vi "_Current Data Global.vi"(4 "error in (no error)":errorcluster, 5 "AcqMethod":T1[](array[typedef]) {"ScanType" format="%#.6g"; "Mass Range"."Res" items=["High/High", "Medium/Medium", "Low/Low", "High/Medium", "High/Low", "Medium/High", "Medium/Low", "Low/High", "Low/Medium"]}, 6 "Spectrum in":i32[](array[numeric]), 7 "Operation":T7=enum."Get Data") -> (0 "error out":errorcluster, 2 "Latest Raw Data":i32[](array[numeric]), 3 "CurrentData":T6[](array[typedef]) {"Method"."Mass Range"."Res" items=["High/High", "Medium/Medium", "Low/Low", "High/Medium", "High/Low", "Medium/High", "Medium/Low", "Low/High", "Low/Medium"]})   [LabVIEW 2015]
uses:
  Type/_Data Operation.ctl
  Type/_Current Data.ctl
  Type/_XML Expt.ctl
  Type/_XML Lens.ctl
  Type/_Mass Range Property.ctl
  Type/_Mass Range Parameters.ctl
  Type/_RT Res Type.ctl
  Type/_Run Module.ctl
  Type/_File Command.ctl
  Configuration/_Global Configuration.vi
panel:
  # "Raw Data:\nExpt#, Run Time in mS, data array in counts"
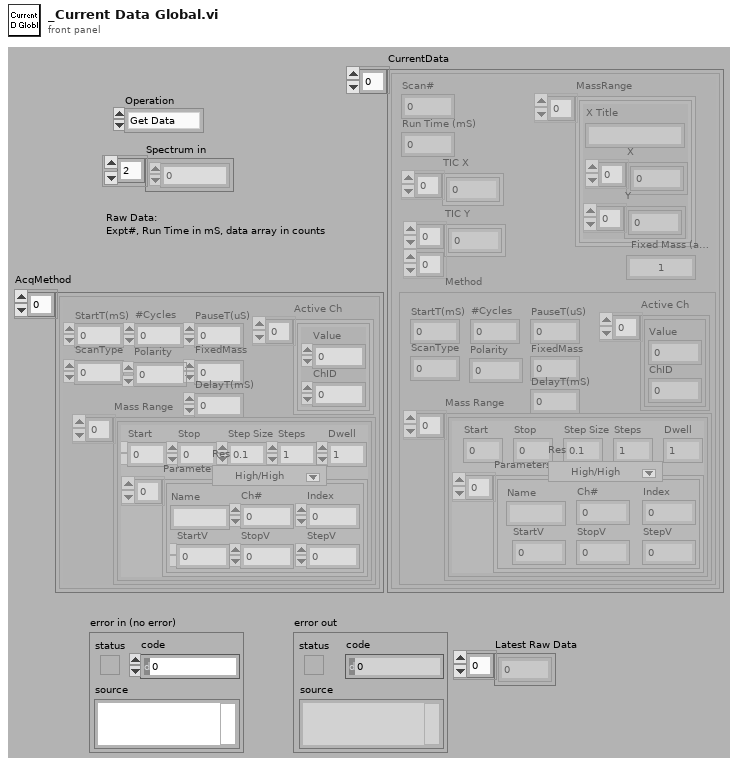
[diagram p1: front panel]
types:
  T1 = typedef "_XML Expt.ctl" = cluster{"StartT(mS)":i32, "#Cycles":i32, "PauseT(uS)":i32, "ScanType":i32, "Polarity":u8, "FixedMass":dbl, "DelayT(mS)":i32, "Active Ch":T2[], "Mass Range":T3[]}
  T2 = typedef "_XML Lens.ctl" = cluster{"Value":dbl, "ChID":u8}
  T3 = typedef "_Mass Range Property.ctl" = cluster{"Start":dbl, "Stop":dbl, "Step Size":dbl, "Steps":i32, "Dwell":dbl, "Parameters":T4[], "Res":T5}
  T4 = typedef "_Mass Range Parameters.ctl" = cluster{"Name":string, "Ch#":u8, "StartV":dbl, "StopV":dbl, "StepV":dbl, "Index":u8}
  T5 = typedef "_RT Res Type.ctl" = u16
  T6 = typedef "_Current Data.ctl" = cluster{"Scan#":i32, "Run Time (mS)":i32, "TIC X":dbl[], "TIC Y":dbl[][], "MassRange":cluster{"X Title":string, "X":dbl[], "Y":i32[]}[], "Fixed Mass (amu)":dbl, "Method":T1}
  T7 = typedef "_Data Operation.ctl" = enum8{"Initialize", "Get Data", "Set Data", "Close"}
  T8 = typedef "_Run Module.ctl" = u16
  T9 = typedef "_File Command.ctl" = enum16{"No Command", "Open", "Open Read", "Write", "Get Spectrum", "Close"}
  T10 = typedef "_Lens Property.ctl" = cluster{"Scan Type":u8, "Scans":i32, "Time 1":dbl, "Time 2":dbl, "Value 1":dbl, "Value 2":dbl, "Step Size":dbl}
  T11 = typedef "_Run Mode.ctl" = enum16{"MRM (Q1/Q2)", "Q1 Scan", "Q1 SRM", "Q2 Scan", "Q2 SRM", "Product Scan", "Precursor Scan", "Neutral Loss", "Neutral Gain"}
  T12 = cluster{"Lenses":T10[], "Mass Ranges":T3[], "Acquire":bool, "MCA":bool, "Q1DC EN":bool, "Q1 POL":bool, "Q3 POL":bool, "Q1 RF  EN":bool, "Averaging":bool, "Log Scale":bool, "CPS":bool, "Unit":bool, "Data Path":path, "Run Mode":T11, "Fixed Mass (amu)":dbl, "Q3DC EN":bool, "Q3 RF  EN":bool, "Negative":bool}
  T13 = cluster{"X Title":string, "X":dbl[], "Y":i32[]}[]
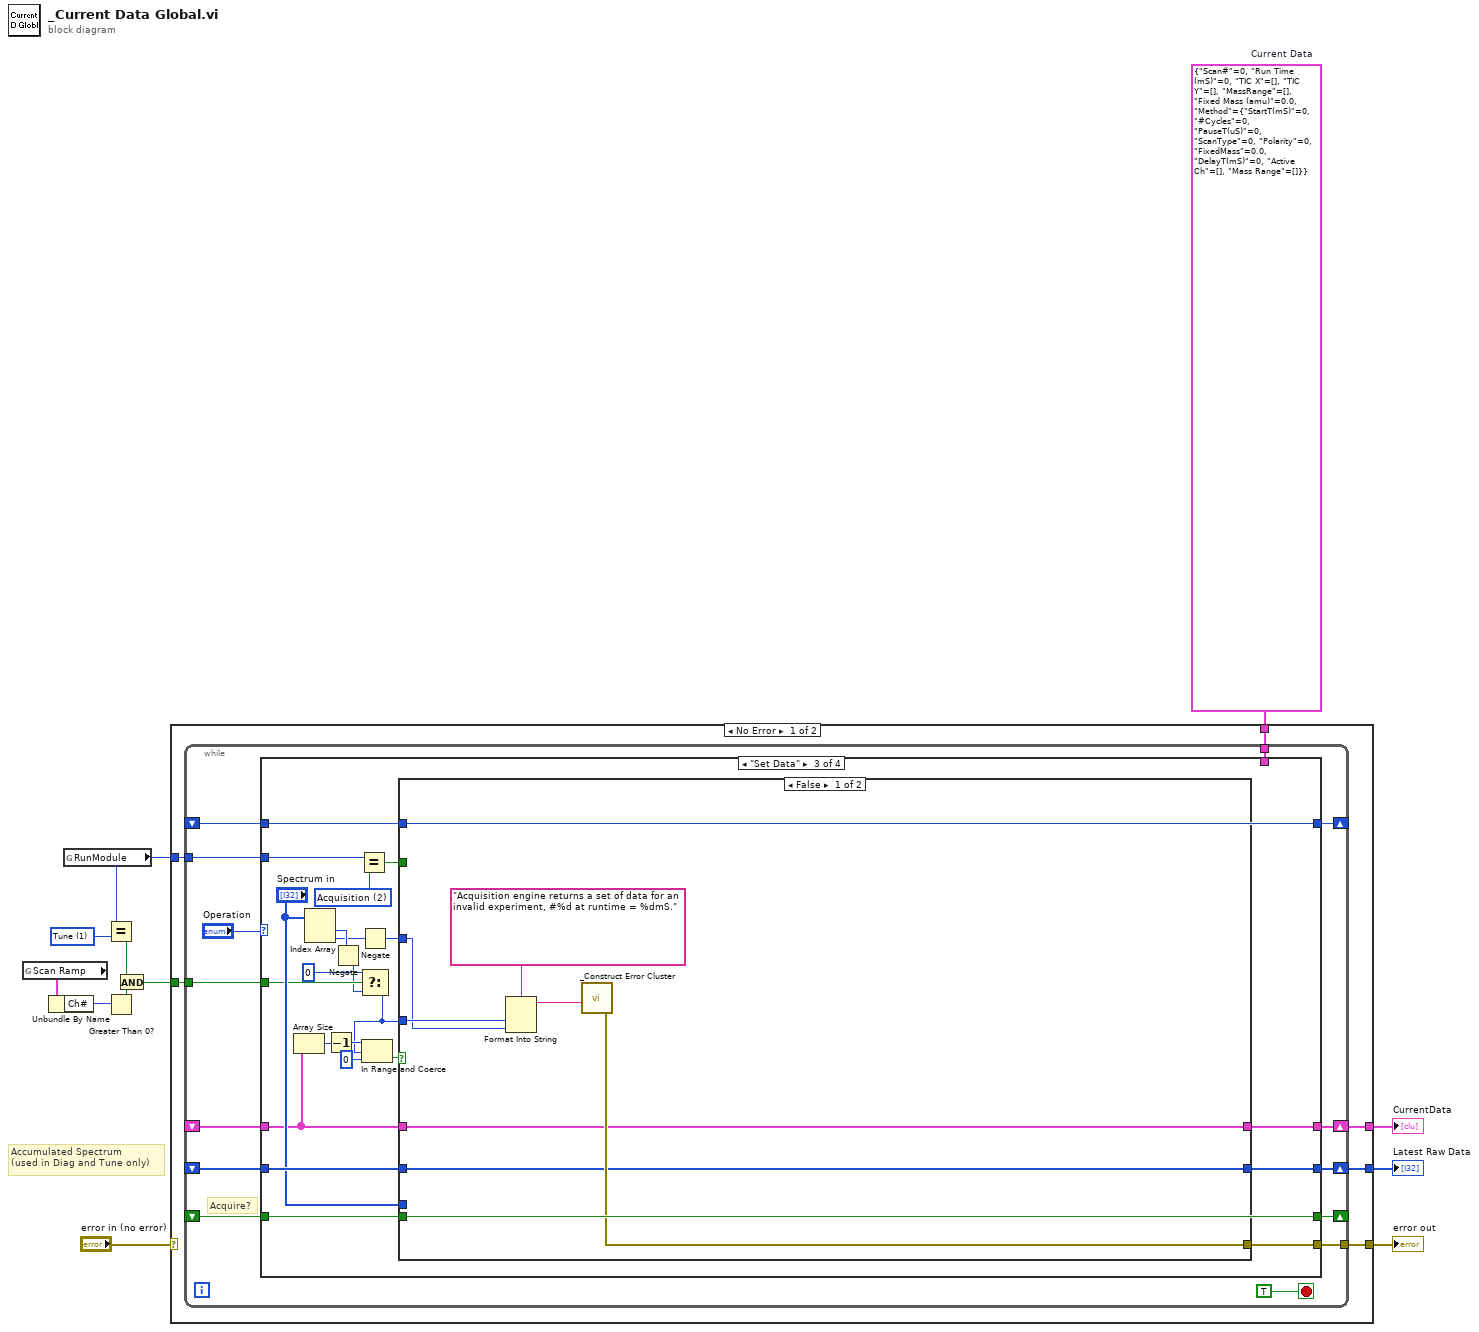
[diagram p0: block diagram]
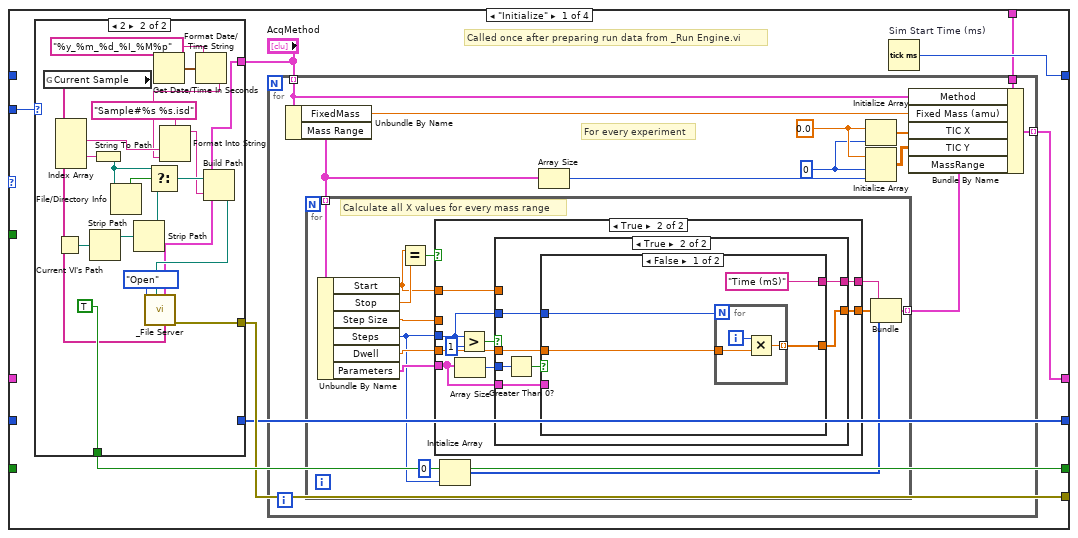
[diagram p2: hidden frame]
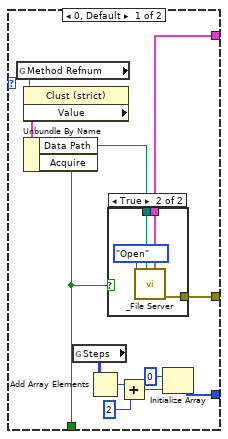
[diagram p3: hidden frame]
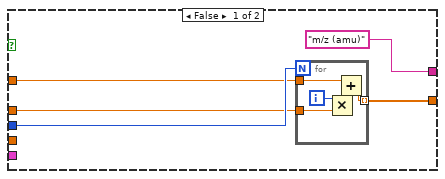
[diagram p5: hidden frame]
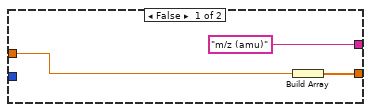
[diagram p6: hidden frame]
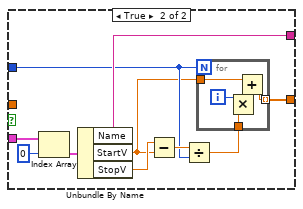
[diagram p7: hidden frame]
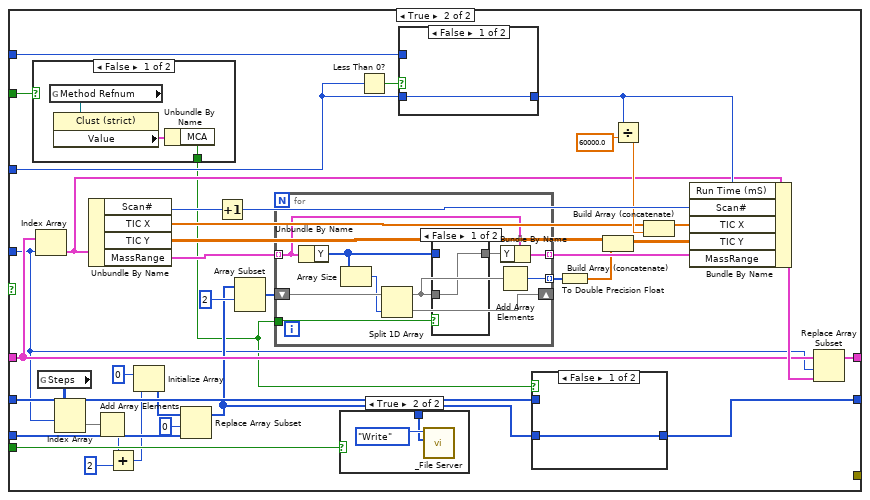
[diagram p9: hidden frame]
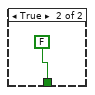
[diagram p10: hidden frame]
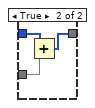
[diagram p11: hidden frame]
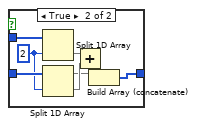
[diagram p12: hidden frame]
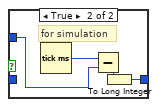
[diagram p14: hidden frame]
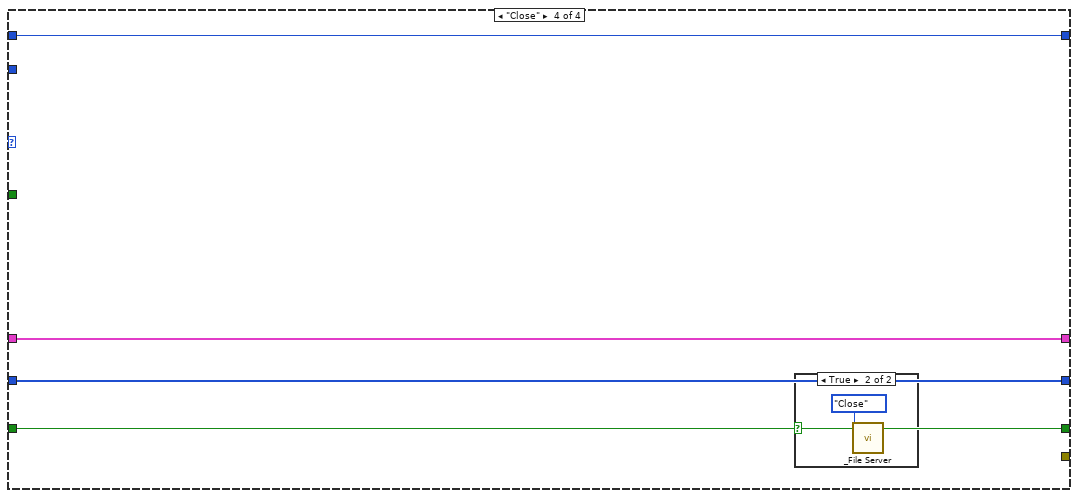
[diagram p15: hidden frame]
diagram:
  w7 = T8 1 items=["Diagnostics", "Tune", "Acquisition"] ("y")
  w9 = T6 {"Scan#"=0, "Run Time (mS)"=0, "TIC X"=[], "TIC Y"=[], "MassRange"=[], "Fixed Mass (amu)"=0.0, "Method"={"StartT(mS)"=0, "#Cycles"=0, "PauseT(uS)"=0, "ScanType"=0, "Polarity"=0, "FixedMass"=0.0, "DelayT(mS)"=0, "Active Ch"=[], "Mass Range"=[]}}  # Current Data
  # "Accumulated Spectrum\n(used in Diag and Tune only)"
  n1 = global read "_Global Configuration.vi" "Scan Ramp"() -> (w6:T4)
  n2 = Unbundle By Name(w6) -> ("Ch#"=w5:u8)
  n3 = global read "_Global Configuration.vi" "RunModule"() -> (w2:T8)
  n4 = Equal?(x=w2, y=w7) -> (x = y?=w4:bool)
  n5 = Greater Than 0?(x=w5) -> (x > 0?=w3:bool)
  n6 = And(x=w4, y=w3) -> (x .and. y?=w1:bool)
  n7 = case shown="No Error" "error in (no error)" {
    selector: "error in (no error)" -> [_ w261]
    tunnel: [w18 _] -> w8
    tunnel: [w17 w261] -> w11
    tunnel: [w16 _] -> w10
    tunnel: w2 -> [w15 _]
    tunnel: w9 -> [w14 _]
    tunnel: w1 -> [w13 _]
    frame No Error {
      n8 = while {
        shift-right: [w30] -> w18
        shift-left: _ -> [w29]
        tunnel: [w28] -> w17
        shift-right: [w27] -> _
        shift-left: _ -> [w26]
        shift-right: [w25] -> w16
        shift-left: _ -> [w24]
        shift-right: [w23] -> _
        shift-left: _ -> [w22]
        tunnel: w15 -> [w21]
        tunnel: w14 -> [w20]
        tunnel: w13 -> [w19]
        stop <- TRUE stop-if-true
        # "Acquire?"
        n9 = case shown="\"Set Data\"" "Operation" {
          tunnel: [w37 w154 w176 w259] -> w30
          tunnel: w29 -> [_ w154 w162 w259]
          tunnel: [w35 _ w165 _] -> w28
          tunnel: [w36 w153 w172 w258] -> w27
          tunnel: w26 -> [_ w153 w172 w258]
          tunnel: [w34 w152 w173 w257] -> w25
          tunnel: w24 -> [_ w152 w174 w257]
          tunnel: [w40 w151 w175 w256] -> w23
          tunnel: w22 -> [_ w151 w175 w256]
          tunnel: w21 -> [w39 _ w161 _]
          tunnel: w20 -> [w38 _ _ _]
          tunnel: w19 -> [_ _ w158 _]
          frame "Initialize" {
            # "Called once after preparing run data from _Run Engine.vi"
            n10 = case shown="2" w39 {
              tunnel: [w49 w72] -> w35
              tunnel: [w48 TRUE] -> w36
              tunnel: [w42 _] -> w34
              tunnel: "AcqMethod" -> [w41 w58]
              frame 0, Default {
                n11 = global read "_Global Configuration.vi" "Method Refnum"() -> (w52:refnum<vi>)
                n12 = property class="Clust (strict)"(reference=w52) -> ("Value"=w51:T12)  [unwired: 1 in, 2 out]
                n13 = Unbundle By Name(w51) -> ("Data Path"=w50:path, "Acquire"=w48:bool)
                n14 = global read "_Global Configuration.vi" "Steps"() -> (w46:i32[][])
                n15 = Add Array Elements(numeric array=w46) -> (sum=w47:i32)
                n16 = case shown="True" w48 {
                  tunnel: [_ w55] -> w49
                  tunnel: w50 -> [_ w54]
                  tunnel: w41 -> [_ w53]
                  frame False {
                  }
                  frame True {
                    n17 = call "_File Server.vi"("AcqMethod"=w53, "file path"=w54, "File Command"=_File_Command."Open") -> ("error out"=w55:errorcluster)  [unwired: 4 in, 4 out]
                  }
                }
                n18 = Add(x=w47, y=2) -> (x+y=w44:i32)
                n19 = Initialize Array(0 ("element"), w44) -> (w42:i32[])
              }
              frame 2 {
                n20 = global read "_Global Configuration.vi" "Current Sample"() -> (w57:string[])
                n21 = Current VI's Path() -> (path=w67:path)
                n22 = Index Array(array=w57) -> (element #1=w71:string, element #3=w75:string)  [unwired: 4 in, 2 out]
                n23 = Strip Path(path=w67) -> (stripped path=w68:path)  [unwired: 1 out]
                n24 = String To Path(string=w75) -> (path=w69:path)
                n25 = File/Directory Info(path=w69) -> (directory=w70:bool)  [unwired: 1 in, 6 out]
                n26 = Strip Path(path=w68) -> (stripped path=w66:path)  [unwired: 1 out]
                n27 = Select(t=w69, s=w70, f=w66) -> (s? t:f=w65:path)
                n28 = Get Date/Time In Seconds() -> (seconds since 1Jan1904=w63:timestamp)
                n29 = Format Date/Time String(time format string (%c)="%y_%m_%d_%I_%M%p", seconds (now)=w63) -> (date/time string=w61:string)  [unwired: 1 out]
                n30 = Format Into String(format string="Sample#%s %s.isd", w71, w61) -> (resulting string=w59:string)  [unwired: 2 in, 1 out]
                n31 = Build Path(base path=w65, name or relative path=w59) -> (appended path=w64:path)
                n32 = call "_File Server.vi"("Sample Info"=w57, "AcqMethod"=w58, "file path"=w64, "File Command"=_File_Command."Open") -> ("error out"=w72:errorcluster)  [unwired: 3 in, 4 out]
              }
            }
            n33 = for {
              tunnel: "AcqMethod" -> [w77] mode=indexing
              tunnel: w38 -> [w86]
              tunnel: [w78] -> w37 mode=indexing
              w81 = 0.0 ("element")
              w76 = 0 ("dimension size")
              # "For every experiment"
              n34 = Unbundle By Name(w77) -> ("FixedMass"=w85:dbl, "Mass Range"=w82:T3[])
              n35 = for {
                tunnel: w82 -> [w99] mode=indexing
                tunnel: [w90] -> w84 mode=indexing
                # "Calculate all X values for every mass range"
                n36 = Unbundle By Name(w99) -> ("Start"=w96:dbl, "Stop"=w97:dbl, "Step Size"=w95:dbl, "Steps"=w87:i32, "Dwell"=w88:dbl, "Parameters"=w89:T4[])
                n37 = Equal?(x=w96, y=w97) -> (x = y?=w98:bool)
                n38 = case shown="True" w98 {
                  tunnel: w87 -> [w104 w111]
                  tunnel: w96 -> [w103 w116]
                  tunnel: w95 -> [w102 _]
                  tunnel: [w101 w114] -> w92
                  tunnel: ["m/z (amu)" ("X Title") w115] -> w93
                  tunnel: w89 -> [_ w110]
                  tunnel: w88 -> [_ w112]
                  frame False {
                    n39 = for {
                      N: w104 -> [_]
                      tunnel: w102 -> [w108]
                      tunnel: w103 -> [w106]
                      tunnel: [w105] -> w101 mode=indexing
                      i -> [w109]
                      n40 = Multiply(x=w109, y=w108) -> (x*y=w107:dbl)
                      n41 = Add(x=w106, y=w107) -> (x+y=w105:dbl)
                    }
                  }
                  frame True {
                    n42 = Array Size(array=w110) -> (size(s)=w113:i32)
                    n43 = Greater?(x=w111, y=1) -> (0:w117:bool)
                    n44 = case shown="True" w117 {
                      tunnel: w116 -> [w119 _]
                      tunnel: ["m/z (amu)" ("X Title") w126] -> w115
                      tunnel: [w120 w123] -> w114
                      tunnel: w113 -> [_ w128]
                      tunnel: w112 -> [_ w125]
                      tunnel: w111 -> [_ w124]
                      tunnel: w110 -> [_ w122]
                      frame False {
                        n45 = Build Array(w119) -> (w120:dbl[])
                      }
                      frame True {
                        n46 = Greater Than 0?(x=w128) -> (x > 0?=w127:bool)
                        n47 = case shown="False" w127 {
                          tunnel: ["Time (mS)" ("X Title") w142] -> w126
                          tunnel: w125 -> [w131 _]
                          tunnel: w124 -> [w130 w139]
                          tunnel: [w129 w136] -> w123
                          tunnel: w122 -> [_ w145]
                          frame False {
                            n48 = for {
                              N: w130 -> [_]
                              tunnel: w131 -> [w134]
                              tunnel: [w133] -> w129 mode=indexing
                              i -> [w135]
                              n49 = Multiply(x=w135, y=w134) -> (x*y=w133:dbl)
                            }
                          }
                          frame True {
                            n50 = Index Array(array=w145, index=0) -> (element=w143:T4)
                            n51 = Unbundle By Name(w143) -> ("Name"=w142:string, "StartV"=w138:dbl, "StopV"=w141:dbl)
                            n52 = Subtract(x=w141, y=w138) -> (x-y=w140:dbl)
                            n53 = Divide(x=w140, y=w139) -> (x/y=w137:dbl)
                            n54 = for {
                              N: w139 -> [_]
                              tunnel: w138 -> [w148]
                              tunnel: [w147] -> w136 mode=indexing
                              tunnel: w137 -> [w146]
                              i -> [w150]
                              n55 = Multiply(x=w150, y=w146) -> (x*y=w149:dbl)
                              n56 = Add(x=w148, y=w149) -> (x+y=w147:dbl)
                            }
                          }
                        }
                      }
                    }
                  }
                }
                n57 = Initialize Array(0 ("element"), w87) -> (w91:i32[])
                n58 = Bundle("Name"=w93, w92, w91) -> (w90:cluster{"Name":string, dbl[], i32[]})  [unwired: 1 out]
              }
              n59 = Array Size(array=w82) -> (size(s)=w83:i32)
              n60 = Initialize Array(w81, w76) -> (w80:dbl[])
              n61 = Initialize Array(w81, w76, w83) -> (w79:dbl[][])
              n62 = Bundle By Name(cluster=w86, "Method"=w77, "Fixed Mass (amu)"=w85, "TIC X"=w80, "TIC Y"=w79, "MassRange"=w84) -> (w78:T6)
            }
            n63 = Tick Count (ms) "Sim Start Time (ms)"() -> (millisecond timer value=w40:u32)
          }
          frame "Get Data", Default {
          }
          frame "Set Data" {
            w160 = T8 2 items=["Diagnostics", "Tune", "Acquisition"] ("y")
            n64 = Array Size(array=w162) -> (size(s)=w169:i32)
            n65 = Index Array(array="Spectrum in") -> (element #1=w170:i32, element #2=w164:i32)  [unwired: 2 in]
            n66 = Decrement(x=w169) -> (x-1=w167:i32)
            n67 = Negate(x=w170) -> (-x=w157:i32)
            n68 = Equal?(x=w161, y=w160) -> (x = y?=w159:bool)
            n69 = Negate(x=w164) -> (-x=w163:i32)
            n70 = Select(t=0, s=w158, f=w157) -> (s? t:f=w155:i32)
            n71 = In Range and Coerce(upper limit=w167, x=w155, lower limit=0) -> (In Range?=w166:bool)  [unwired: 1 out]
            n72 = case shown="False" w166 {
              tunnel: w163 -> [w179 w199]
              tunnel: [w178 w195] -> w176
              tunnel: w175 -> [_ w221]
              tunnel: w174 -> [w177 w220]
              tunnel: [w177 w219] -> w173
              tunnel: w172 -> [_ w218]
              tunnel: "Spectrum in" -> [_ w217]
              tunnel: w155 -> [w183 w192]
              tunnel: [w180 _] -> w165
              tunnel: w162 -> [w178 w196]
              tunnel: w159 -> [_ w185]
              frame False {
                n73 = Format Into String(format string="Acquisition engine returns a set of data for an invalid experiment, #%d at runtime = %dmS.", w183, w179) -> (resulting string=w181:string)  [unwired: 2 in, 1 out]
                n74 = call "_Construct Error Cluster.vi"("reason"=w181) -> ("error out"=w180:errorcluster)  [unwired: 3 in, 3 out]
              }
              frame True {
                n75 = case shown="False" w185 {
                  tunnel: [w222 FALSE] -> w184
                  frame False {
                    n76 = global read "_Global Configuration.vi" "Method Refnum"() -> (w223:refnum<vi>)
                    n77 = property class="Clust (strict)"(reference=w223) -> ("Value"=w224:T12)  [unwired: 1 in, 2 out]
                    n78 = Unbundle By Name(w224) -> ("MCA"=w222:bool)
                  }
                  frame True {
                  }
                }
                n79 = Index Array(array=w196, index=w192) -> (element=w198:T6)
                n80 = global read "_Global Configuration.vi" "Steps"() -> (w193:i32[][])
                n81 = Index Array(array=w193, index (row)=w192) -> (element=w191:i32[])  [unwired: 1 in]
                n82 = Unbundle By Name(w198) -> ("Scan#"=w215:i32, "TIC X"=w209:dbl[], "TIC Y"=w202:dbl[][], "MassRange"=w206:T13)
                n83 = Add Array Elements(numeric array=w191) -> (sum=w190:i32)
                n84 = Add(x=w190, y=2) -> (x+y=w188:i32)
                n85 = Initialize Array(0 ("element"), w188) -> (w186:i32[])
                n86 = Replace Array Subset(array=w186, new element=w217, index=0) -> (w194:i32[])
                n87 = Increment(x=w215) -> (x+1=w214:i32)
                n88 = Array Subset(array=w194, index=2) -> (w205:i32[])  [unwired: 1 in]
                n89 = for {
                  tunnel: w206 -> [w233] mode=indexing
                  shift-right: [w227] -> _
                  shift-left: w205 -> [w235]
                  tunnel: [w232] -> w204 mode=indexing
                  tunnel: w184 -> [w231]
                  tunnel: [w226] -> w203 mode=indexing
                  n90 = Unbundle By Name(w233) -> ("Y"=w230:i32[])
                  n91 = Array Size(array=w230) -> (size(s)=w234:i32)
                  n92 = Split 1D Array(array=w235, index=w234) -> (first subarray=w228:i32[], second subarray=w227:i32[])
                  n93 = case shown="False" w231 {
                    tunnel: w228 -> [w236 w238]
                    tunnel: w230 -> [_ w239]
                    tunnel: [w236 w237] -> w229
                    frame False {
                    }
                    frame True {
                      n94 = Add(x=w239, y=w238) -> (x+y=w237:i32[])
                    }
                  }
                  n95 = Add Array Elements(numeric array=w228) -> (sum=w226:i32)
                  n96 = Bundle By Name(cluster=w233, "Y"=w229) -> (w232:cluster{"X Title":string, "X":dbl[], "Y":i32[]})
                }
                n97 = case shown="True" w218 {
                  tunnel: w194 -> [_ w249]
                  frame False {
                  }
                  frame True {
                    n98 = call "_File Server.vi"("Spectrum"=w249, "File Command"=_File_Command."Write") -> ()  [unwired: 5 in, 5 out]
                  }
                }
                n99 = Less Than 0?(x=w199) -> (x < 0?=w216:bool)
                n100 = case shown="False" w216 {
                  tunnel: w199 -> [w251 _]
                  tunnel: [w251 w254] -> w211
                  tunnel: w221 -> [_ w252]
                  frame False {
                  }
                  frame True {
                    # "for simulation"
                    n101 = Tick Count (ms)() -> (millisecond timer value=w255:u32)
                    n102 = Subtract(x=w255, y=w252) -> (x-y=w253:u32)
                    n103 = To Long Integer(number=w253) -> (32bit integer=w254:i32)
                  }
                }
                n104 = case shown="False" w184 {
                  tunnel: [w240 w243] -> w219
                  tunnel: w194 -> [w240 w248]
                  tunnel: w220 -> [_ w241]
                  frame False {
                  }
                  frame True {
                    w247 = 2 ("index")
                    n105 = Split 1D Array(array=w241, index=w247) -> (second subarray=w246:i32[])  [unwired: 1 out]
                    n106 = Split 1D Array(array=w248, index=w247) -> (first subarray=w242:i32[], second subarray=w245:i32[])
                    n107 = Add(x=w246, y=w245) -> (x+y=w244:i32[])
                    n108 = Build Array (concatenate)(w242, w244) -> (w243:i32[])
                  }
                }
                n109 = To Double Precision Float(number=w203) -> (double precision float=w201:dbl[])
                n110 = Build Array (concatenate)(w202, w201) -> (w200:dbl[][])
                n111 = Divide(x=w211, y=60000.0) -> (x/y=w210:dbl)
                n112 = Build Array (concatenate)(w209, w210) -> (w208:dbl[])
                n113 = Bundle By Name(cluster=w198, "Run Time (mS)"=w211, "Scan#"=w214, "TIC X"=w208, "TIC Y"=w200, "MassRange"=w204) -> (w197:T6)
                n114 = Replace Array Subset(array=w196, new element=w197, index=w192) -> (w195:T6[])
              }
            }
          }
          frame "Close" {
            n115 = case shown="True" w258 {
              frame False {
              }
              frame True {
                n116 = call "_File Server.vi"("File Command"=_File_Command."Close") -> ()  [unwired: 6 in, 5 out]
              }
            }
          }
        }
      }
    }
    frame Error {
    }
  }
  "error out" <- w11
  "Latest Raw Data" <- w10
  "CurrentData" <- w8
